vi "sutter_driver.vi"() -> ()   [LabVIEW 2014]
uses:
  <vilib>/Instr/_visa.llb/VISA Configure Serial Port (Instr).vi
panel:
  out "Boolean":bool
  out "Numeric":i32
  out "error out 2":errorcluster
  in  "y":cluster{"Go Home":bool, "Position":dbl[]}[](array[cluster])
  in  "Motor Poisition":dbl[][](array[numeric]) caption="Motor Poisition\nA               B"
  in  "error in (no error)":errorcluster
  in  "stop":bool
  in  "VISA resource name":refnum<visa-resource-name>
  # "Motor Poisition\nA               B"
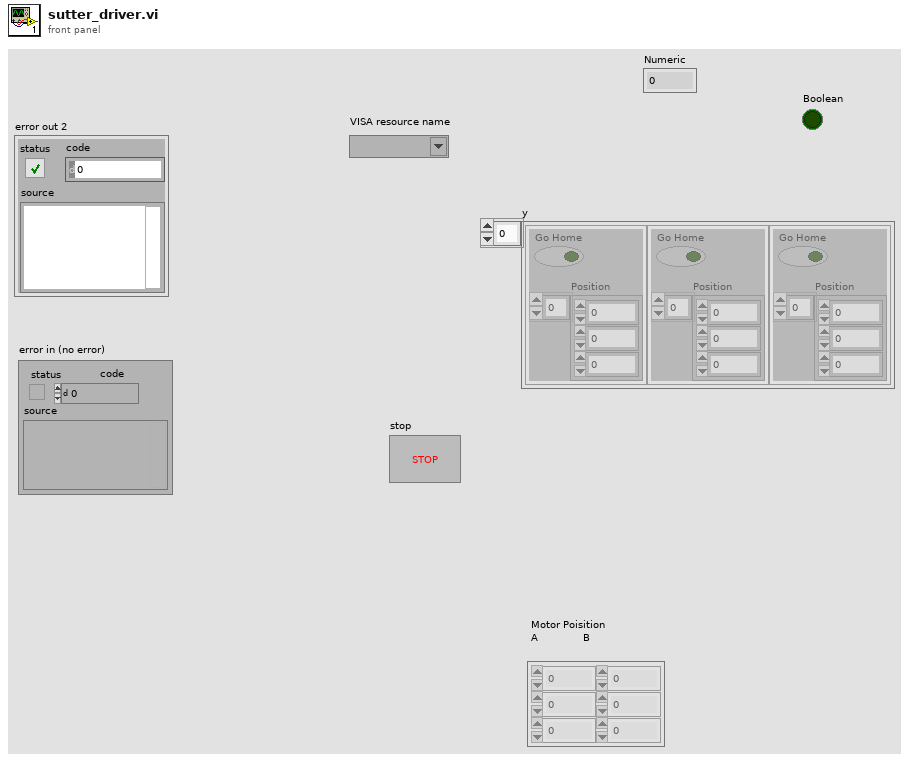
[diagram p1: front panel]
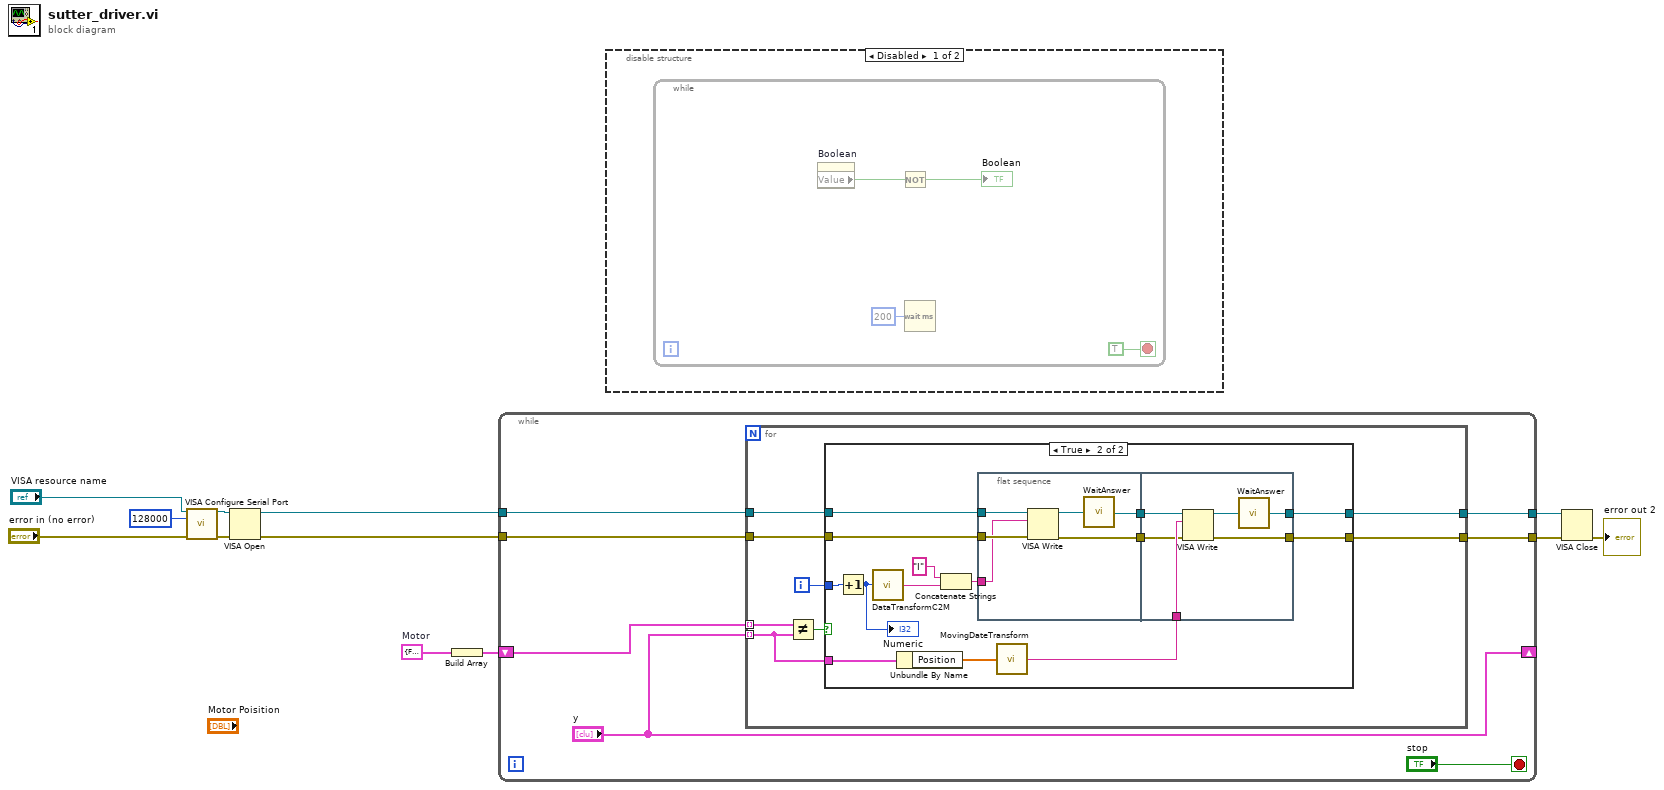
[diagram p0: block diagram]
diagram:
  w5 = cluster{"Go Home":bool, "Position":dbl[]} {"Go Home"=FALSE, "Position"=[0.0, 0.0, 0.0]}  # Motor
  n1 = call-poly "VISA Configure Serial Port"("VISA resource name"="VISA resource name", "baud rate (9600)"=u32 128000, "error in (no error)"="error in (no error)") -> ("VISA resource name out"=w10:refnum<visa-resource-name>, "error out"=w8:errorcluster)  [unwired: 11 in]
  n2 = VISA Open(error in (no error)=w8, VISA resource name=w10) -> (VISA resource name=w7:refnum<visa-resource-name>, error out=w6:errorcluster)  [unwired: 3 in]
  n3 = Build Array(w5) -> (w4:cluster{"Go Home":bool, "Position":dbl[]}[])
  n4 = while {
    tunnel: w7 -> [w18]
    tunnel: w6 -> [w17]
    shift-right: ["y"] -> _
    shift-left: w4 -> [w19]
    tunnel: [w14] -> w2
    tunnel: [w13] -> w1
    stop <- "stop" stop-if-true
    n5 = for {
      tunnel: w19 -> [w27] mode=indexing
      tunnel: "y" -> [w22] mode=indexing
      tunnel: w18 -> [w25]
      tunnel: w17 -> [w23]
      tunnel: [w21] -> w14
      tunnel: [w20] -> w13
      i -> [w24]
      n6 = Not Equal?(x=w27, y=w22) -> (x != y?=w26:bool)
      n7 = case shown="True" w26 {
        tunnel: w25 -> [w29 w43]
        tunnel: w24 -> [_ w31]
        tunnel: w23 -> [w28 w42]
        tunnel: w22 -> [_ w41]
        tunnel: [w29 w33] -> w21
        tunnel: [w28 w32] -> w20
        frame False {
        }
        frame True {
          n8 = Increment(x=w31) -> (x+1=w30:i32)
          "Numeric" <- w30
          n9 = call "DataTransformC2M.vi"("input"=w30) -> ("output"=w35:string)
          n10 = Unbundle By Name(w41) -> ("Position"=w40:dbl[])
          n11 = Concatenate Strings("I" ("string"), w35) -> (w34:string)
          n12 = flat-sequence {
            tunnel: w43 -> [w46]
            tunnel: w42 -> [w49]
            tunnel: [w48] -> w39
            tunnel: [w47] -> w37
            tunnel: w34 -> [w44]
            tunnel: w39 -> [w54]
            tunnel: w38 -> [w53]
            tunnel: w37 -> [w52]
            tunnel: [w51] -> w33
            tunnel: [w50] -> w32
            frame #0 {
              n13 = VISA Write(VISA resource name=w46, write buffer=w44, error in (no error)=w49) -> (VISA resource name out=w45:refnum<visa-resource-name>, error out=w47:errorcluster)  [unwired: 1 out]
              n14 = call "WaitAnswer.vi"("VISA resource name in"=w45) -> ("VISA resource name out"=w48:refnum<visa-resource-name>)
            }
            frame #1 {
              n15 = VISA Write(VISA resource name=w54, write buffer=w53, error in (no error)=w52) -> (VISA resource name out=w55:refnum<visa-resource-name>, error out=w50:errorcluster)  [unwired: 1 out]
              n16 = call "WaitAnswer.vi"("VISA resource name in"=w55) -> ("VISA resource name out"=w51:refnum<visa-resource-name>)
            }
          }
          n17 = call "MovingDateTransform.vi"("INPUT"=w40) -> ("MOVEING COMMAND"=w38:string)  [unwired: 2 in]
        }
      }
    }
  }
  n18 = disable-structure shown="Disabled" {
    frame Disabled {
      n19 = while {
        stop <- TRUE stop-if-true
        n20 = property on="Boolean" class="Bool (strict)"() -> ("Value"=w58:bool)  [unwired: 2 in, 2 out]
        n21 = Not(x=w58) -> (.not. x?=→"Boolean":bool)
        n22 = Wait (ms)(milliseconds to wait=u32 200) -> ()  [unwired: 1 out]
      }
    }
    frame Enabled {
    }
  }
  n23 = VISA Close(VISA resource name=w2, error in (no error)=w1) -> (error out=→"error out 2":errorcluster)
